vi "Search DQMH Module name from selection.vi"(11 "Search Module Name":string="\\Panther Dashboard for DQMH.lvproj\\Coins.lvlib\\Broadcast\\Error Reported") -> (0 "Broadcast?":bool, 3 "Module Name":string)   [LabVIEW 2019, in "Panther Dashboard.lvlib"]
uses:
  Panther Dashboard.lvlib
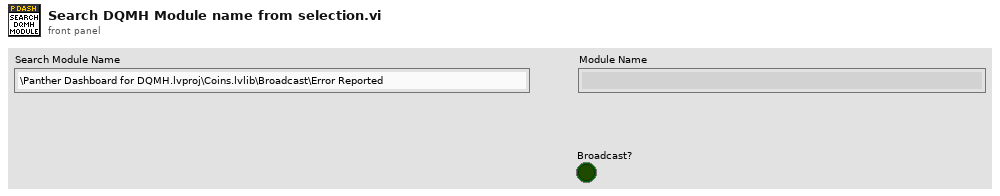
[diagram p1: front panel]
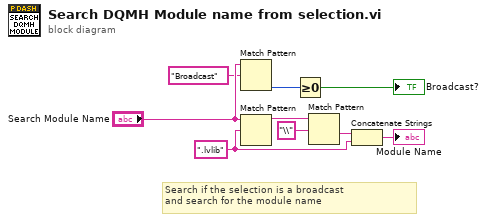
[diagram p0: block diagram]
diagram:
  w9 = ".lvlib" ("regular expression")
  # "Search if the selection is a broadcast\nand search for the module name"
  n1 = Match Pattern(string="Search Module Name", regular expression="Broadcast") -> (offset past match=w2:i32)  [unwired: 1 in, 3 out]
  n2 = Match Pattern(string="Search Module Name", regular expression=w9) -> (before substring=w7:string)  [unwired: 1 in, 3 out]
  n3 = Greater Or Equal To 0?(x=w2) -> (x >= 0?=→"Broadcast?":bool)
  n4 = Match Pattern(string=w7, regular expression="\\") -> (after substring=w5:string)  [unwired: 1 in, 3 out]
  n5 = Concatenate Strings(w5, w9) -> (→"Module Name":string)
